vi "Aplicaderiva1.vi"() -> ()   [LabVIEW 2010]
uses:
  <vilib>/Analysis/NI_AALPro.lvlib
panel:
  out "Waveform Chart":dbl[](graph)
  out "Contagem":i32
  out "Waveform Chart 2":waveform(dbl)(graph)
  in  "Número":i32
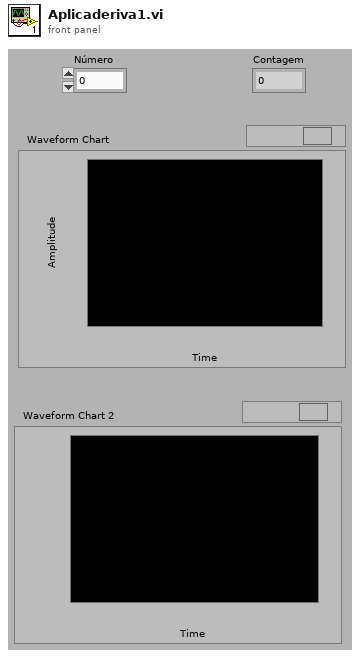
[diagram p1: front panel]
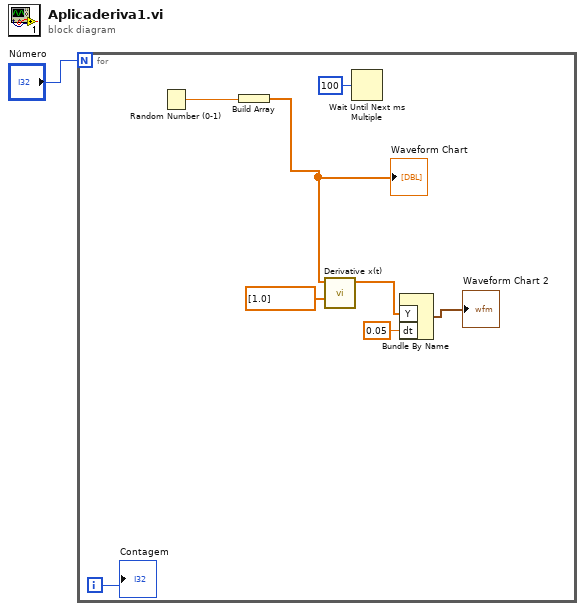
[diagram p0: block diagram]
diagram:
  n1 = for {
    N: "Número" -> [_]
    i -> [w4]
    n2 = Random Number (0-1)() -> (number: 0 to 1=w3:dbl)
    n3 = Build Array(w3) -> (w2:dbl[])
    "Waveform Chart" <- w2
    n4 = call <vilib>:"Derivative x(t).vi"("Final Condition"=dbl[] [1.0], "X"=w2) -> ("dX/dt"=w5:dbl[])  [unwired: 8 in, 1 out]
    n5 = Wait Until Next ms Multiple(millisecond multiple=u32 100) -> ()  [unwired: 1 out]
    n6 = Bundle By Name("Y"=w5, "dt"=0.05) -> (→"Waveform Chart 2":waveform(dbl))  [unwired: 1 in]
    "Contagem" <- w4
  }
